vi "Write Launch Rooms Manager Msg.vi"(10 "Hotel Management Tool UI.lvlib:Launch Rooms Manager Msg.lvclass":refnum<class "Launch Rooms Manager Msg.lvclass">, 11 "Hotel Management Tool UI in":refnum<class "Hotel Management Tool UI.lvclass">) -> (3 "Hotel Management Tool UI out":refnum<class "Hotel Management Tool UI.lvclass">)   [LabVIEW 2023, in "Hotel Management Tool UI.lvlib" / "Hotel Management Tool UI.lvclass"]
uses:
  Hotel Management Tool UI.lvclass
  Hotel Management Tool UI Messages/Launch Rooms Manager Msg/Launch Rooms Manager Msg.lvclass
  Hotel Management Tool UI.lvclass/Hotel Management Tool UI.ctl
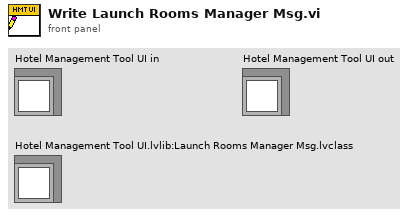
[diagram p1: front panel]
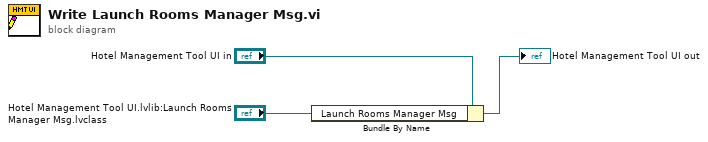
[diagram p0: block diagram]
diagram:
  n1 = Bundle By Name(cluster="Hotel Management Tool UI in", "Launch Rooms Manager Msg"="Hotel Management Tool UI.lvlib:Launch Rooms Manager Msg.lvclass") -> (→"Hotel Management Tool UI out":refnum<class "Hotel Management Tool UI.lvclass">)
